vi "DE_Init Stopping State.vi"(11 "stopping criteria":T2={"max iterations"=50, "max function calls"=-1, "max time (sec)"=-1.0}) -> (3 "stopping state":T1={"max iterations"=50, "max function calls"=-1, "max time (sec)"=-1.0, "cur function calls"=0, "init tick count"=0})   [LabVIEW 2017, in "NI_AAL_GlobalOptimization.lvlib"]
uses:
  <vilib>/gmath/NI_AAL_GlobalOptimization.lvlib
  <vilib>/gmath/GlobalOptimization.llb/DE_Stopping Criteria.ctl
  <vilib>/gmath/GlobalOptimization.llb/DE_Stopping State.ctl
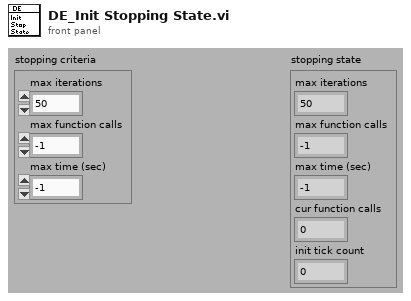
[diagram p1: front panel]
types:
  T1 = typedef "NI_AAL_GlobalOptimization.lvlib/DE_Stopping State.ctl" = cluster{"max iterations":i32, "max function calls":i32, "max time (sec)":dbl, "cur function calls":i32, "init tick count":u32}
  T2 = typedef "NI_AAL_GlobalOptimization.lvlib/DE_Stopping Criteria.ctl" = cluster{"max iterations":i32, "max function calls":i32, "max time (sec)":dbl}
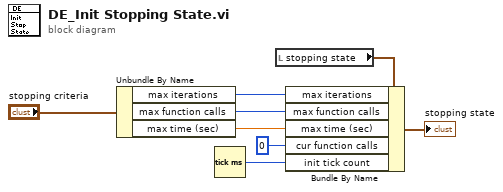
[diagram p0: block diagram]
diagram:
  n1 = Unbundle By Name("stopping criteria") -> ("max iterations"=w6:i32, "max function calls"=w5:i32, "max time (sec)"=w4:dbl)
  n2 = Tick Count (ms)() -> (millisecond timer value=w1:u32)
  n3 = local read "stopping state"() -> (w7:T1)
  n4 = Bundle By Name(cluster=w7, "max iterations"=w6, "max function calls"=w5, "max time (sec)"=w4, "cur function calls"=0, "init tick count"=w1) -> (→"stopping state":T1)
